vi "FactorPass.vi"(7 "Coordenada bola":dbl[](array[numeric]), 8 "geometry":T6, 9 "Coordenada robo":dbl[](array[numeric]), 10 "enemy_robots":T1[](array[typedef]), 11 "enemy_goalie_id":dbl) -> (0 "id inimigo \nmaior diferença \nde tempo":dbl, 1 "Dif. tempo\ninimigo bola":dbl, 2 "t":dbl, 3 "Critério de marcação Normalizado":dbl, 4 "Robô marcado?":bool=TRUE, 5 "Array out":dbl[][](array[numeric]), 6 "menor dist":dbl)   [LabVIEW 2018]
uses:
  newpass/SSLView/Core/Field Size.ctl
  newpass/SSLView/Core/AI Robot.ctl
  newpass/SSLView/Intel/Functions Enum.ctl
  newpass/SSLView/Intel/AttackerStates.ctl
  newpass/SSLView/Path Planning/RRT/PathDests.ctl
  newpass/SSLView/Path Planning/RRT/PathDest.ctl
  2b1c05b2-3bf1-4219-9740-877ec4118c70.vi
  <vilib>/Array/Sort 2D Array - Pop Stack.vi
  <vilib>/Array/Sort 2D Array - Push Stack.vi
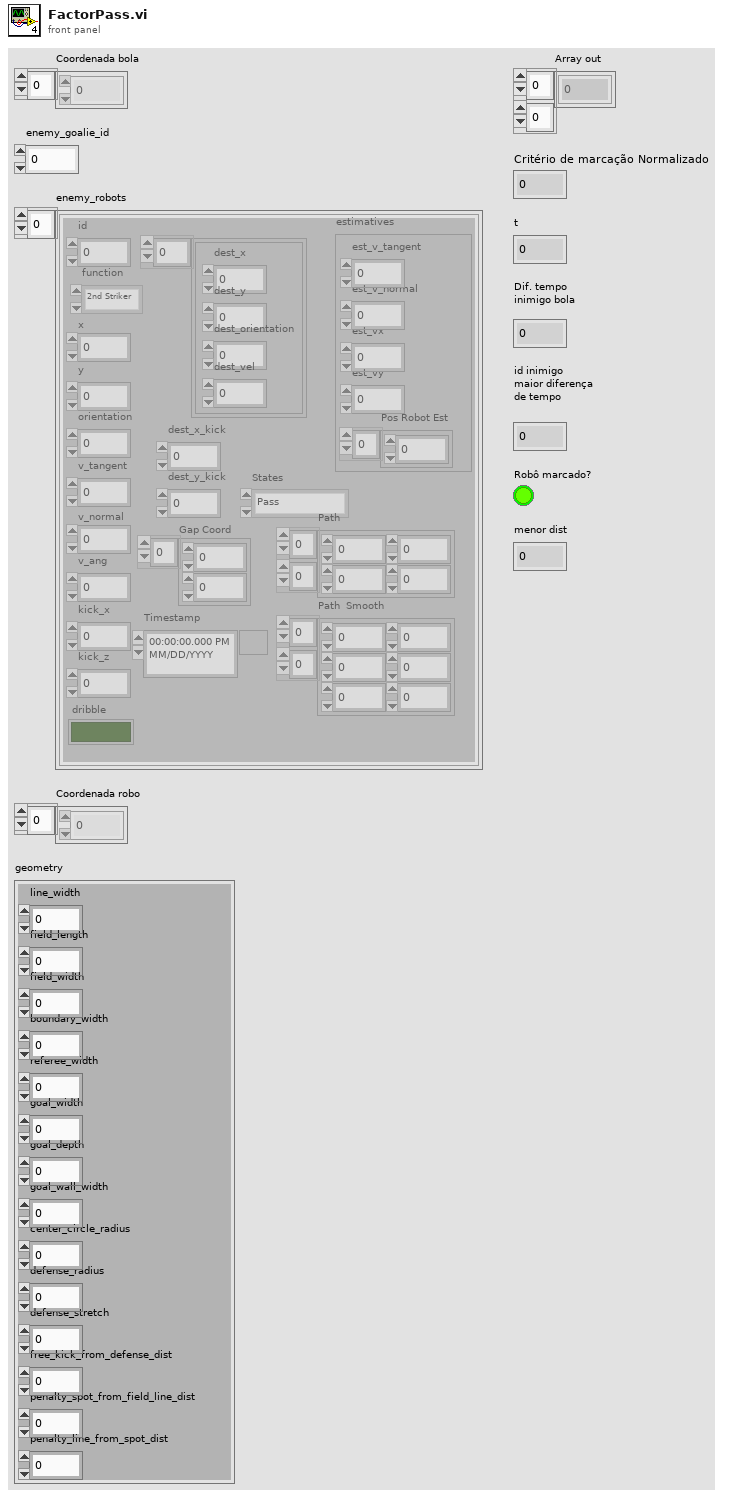
[diagram p1: front panel]
types:
  T1 = typedef "AI Robot.ctl" = cluster{"id":u32, "function":T2, "x":dbl, "y":dbl, "orientation":dbl, "v_tangent":dbl, "v_normal":dbl, "v_ang":dbl, "kick_x":dbl, "kick_z":dbl, "dribble":bool, "Timestamp":timestamp, "estimatives":cluster{"est_v_tangent":dbl, "est_v_normal":dbl, "est_vx":dbl, "est_vy":dbl, "Pos Robot Est":dbl[]}, "dest_x_kick":dbl, "dest_y_kick":dbl, "Gap Coord":dbl[], "States":T3, "Path ":dbl[][], "Path  Smooth":dbl[][], "Dest":T4}
  T2 = typedef "Functions Enum.ctl" = enum16{"2nd Striker", "Attacker", "Goalie", "Defender", "Striker", "Goto 0", "Dummy", "Kicker", "ZigZag 0", "ZigZag 1", "ZigZag 2", "ZigZag 3", "ZigZag 4", "ZigZag 5", "ZigZag 6", "ZigZag 7", "ZigZag 8", ""}
  T3 = typedef "AttackerStates.ctl" = enum16{"Pass", "GoToTangent", "BallGetting", "GoToKick", ""}
  T4 = typedef "PathDests.ctl" = T5[]
  T5 = typedef "PathDest.ctl" = cluster{"dest_x":dbl, "dest_y":dbl, "dest_orientation":dbl, "dest_vel":dbl}
  T6 = typedef "Field Size.ctl" = cluster{"line_width":u32, "field_length":u32, "field_width":u32, "boundary_width":u32, "referee_width":u32, "goal_width":u32, "goal_depth":u32, "goal_wall_width":u32, "center_circle_radius":u32, "defense_radius":u32, "defense_stretch":u32, "free_kick_from_defense_dist":u32, "penalty_spot_from_field_line_dist":u32, "penalty_line_from_spot_dist":u32}
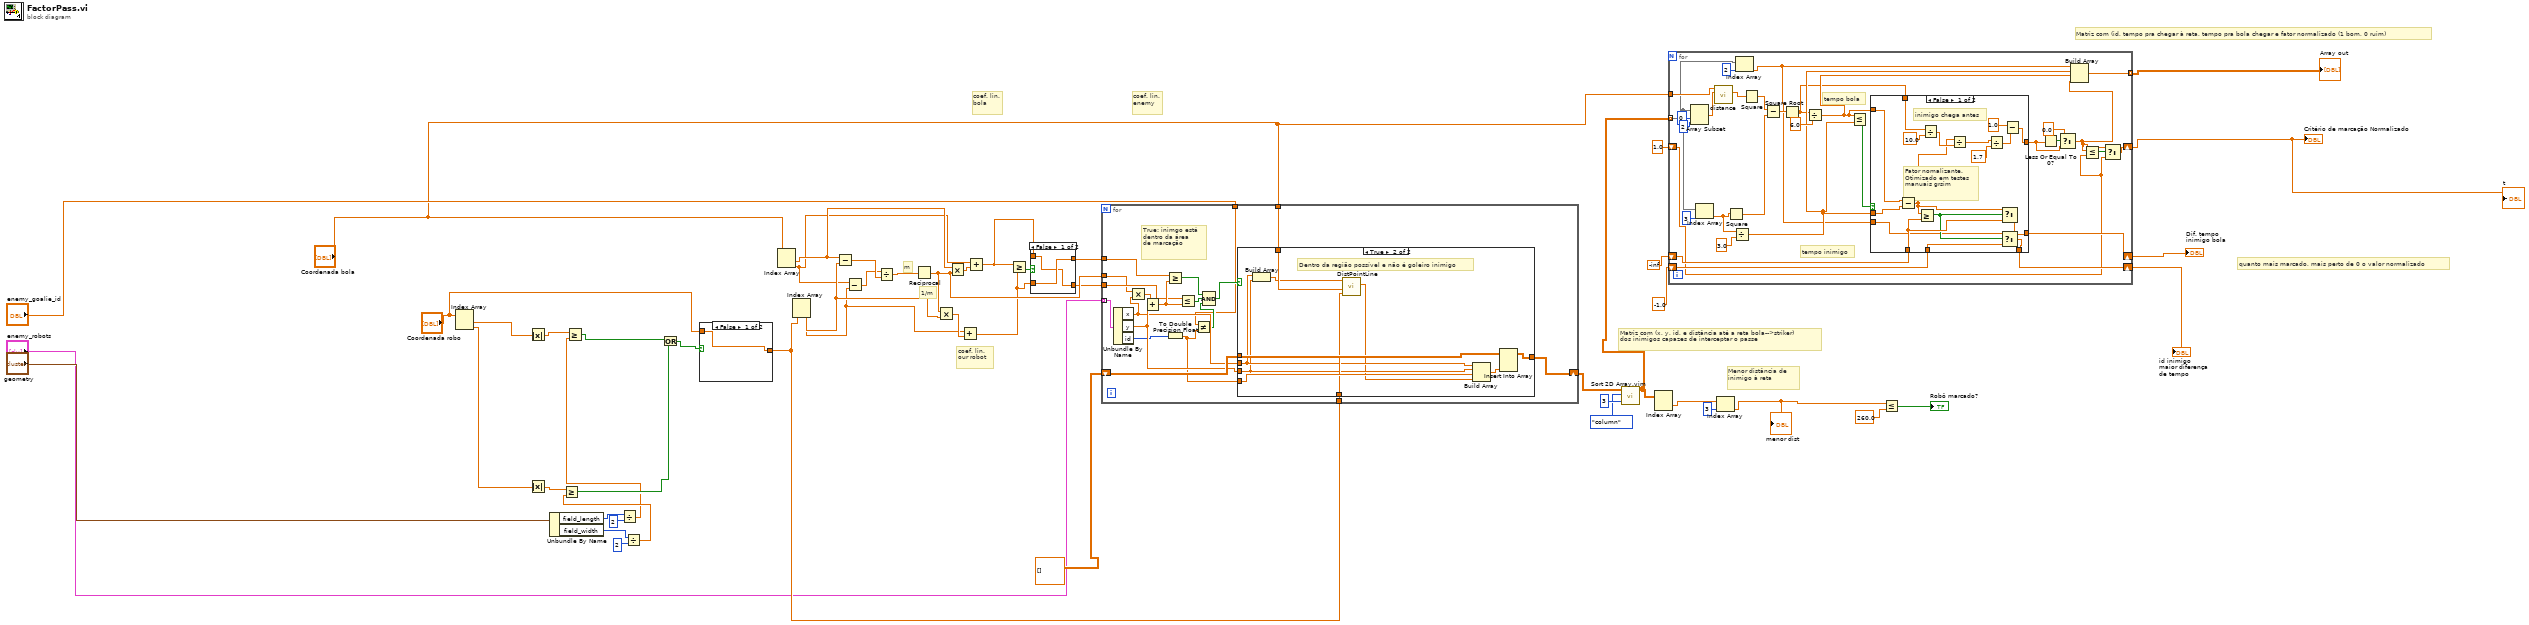
[diagram p0: block diagram]
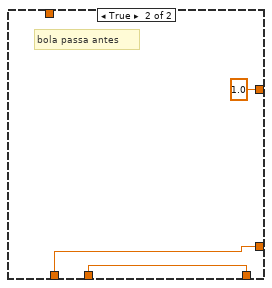
[diagram p2: hidden frame]
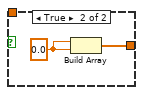
[diagram p3: hidden frame]
diagram:
  # "Matriz com (id, tempo pra chegar à reta, tempo pra bola chegar e fator normalizado (1 bom, 0 ruim)"
  # "quanto mais marcado, mais perto de 0 o valor normalizado"
  # "Menor distância de \ninimigo à reta"
  # "Matriz com (x, y, id, e distância até a reta bola-->striker) \ndos inimigos capazes de interceptar o passe"
  # "coef. lin.\nbola"
  # "coef. lin.\nenemy"
  # "coef. lin.\nour robot"
  # "1/m"
  # "m"
  n1 = Index Array(array="Coordenada robo") -> (element #1=w45:dbl, element #2=w46:dbl)  [unwired: 2 in]
  n2 = Absolute Value(x=w45) -> (abs(x)=w23:dbl)
  n3 = Absolute Value(x=w46) -> (abs(x)=w25:dbl)
  n4 = Unbundle By Name("geometry") -> ("field_length"=w19:u32, "field_width"=w22:u32)
  n5 = Divide(x=w19, y=2) -> (x/y=w24:dbl)
  n6 = Greater Or Equal?(x=w23, y=w24) -> (x >= y?=w27:bool)
  n7 = Divide(x=w22, y=u32 2) -> (x/y=w26:dbl)
  n8 = Greater Or Equal?(x=w25, y=w26) -> (x >= y?=w28:bool)
  n9 = Or(x=w27, y=w28) -> (x .or. y?=w30:bool)
  n10 = case shown="False" w30 {
    tunnel: [w52 w53] -> w31
    tunnel: "Coordenada robo" -> [w52 _]
    frame False {
    }
    frame True {
      w54 = 0.0
      n11 = Build Array(w54, w54) -> (w53:dbl[])
    }
  }
  n12 = Index Array(array="Coordenada bola") -> (element #1=w42:dbl, element #2=w2:dbl)  [unwired: 2 in]
  n13 = Index Array(array=w31) -> (element #1=w41:dbl, element #2=w3:dbl)  [unwired: 2 in]
  n14 = Subtract(x=w42, y=w41) -> (x-y=w5:dbl)
  n15 = Subtract(x=w2, y=w3) -> (x-y=w4:dbl)
  n16 = Divide(x=w4, y=w5) -> (x/y=w1:dbl)
  n17 = Reciprocal(x=w1) -> (1/x=w44:dbl)
  n18 = Multiply(x=w44, y=w41) -> (x*y=w40:dbl)
  n19 = Multiply(x=w42, y=w44) -> (x*y=w43:dbl)
  n20 = Add(x=w3, y=w40) -> (x+y=w9:dbl)
  n21 = Add(x=w2, y=w43) -> (x+y=w8:dbl)
  n22 = Greater Or Equal?(x=w8, y=w9) -> (x >= y?=w7:bool)
  n23 = case shown="False" w7 {
    tunnel: [w56 w58] -> w10
    tunnel: w8 -> [w55 w58]
    tunnel: [w55 w57] -> w11
    tunnel: w9 -> [w56 w57]
    frame False {
    }
    frame True {
    }
  }
  n24 = for {
    tunnel: "enemy_robots" -> [w77] mode=indexing
    tunnel: w44 -> [w65]
    shift-right: [w75] -> w14
    shift-left: dbl[][] [] -> [w76]
    tunnel: w10 -> [w70]
    tunnel: w11 -> [w69]
    tunnel: "Coordenada bola" -> [w67]
    tunnel: w31 -> [w66]
    tunnel: "enemy_goalie_id" -> [w60]
    # "True: inimgo está \ndentro da área\nde marcação"
    n25 = Unbundle By Name(w77) -> ("x"=w64:dbl, "y"=w68:dbl, "id"=w62:u32)
    n26 = Multiply(x=w65, y=w64) -> (x*y=w63:dbl)
    n27 = Add(x=w63, y=w68) -> (x+y=w74:dbl)
    n28 = Greater Or Equal?(x=w70, y=w74) -> (x >= y?=w72:bool)
    n29 = To Double Precision Float(number=w62) -> (double precision float=w59:dbl)
    n30 = Less Or Equal?(x=w69, y=w74) -> (x <= y?=w73:bool)
    n31 = Not Equal?(x=w60, y=w59) -> (x != y?=w61:bool)
    n32 = Compound Arithmetic op=AND(w72, w73, w61) -> (w71:bool)
    n33 = case shown="True" w71 {
      tunnel: w76 -> [w78 w88]
      tunnel: [w78 w87] -> w75
      tunnel: w64 -> [_ w82]
      tunnel: w68 -> [_ w81]
      tunnel: w59 -> [_ w86]
      tunnel: w67 -> [_ w84]
      tunnel: w66 -> [_ w83]
      frame False {
        # "Fora da região possível ou é goleiro inimigo"
      }
      frame True {
        # "Dentro da região possível e não é goleiro inimigo"
        n34 = Build Array(w82, w81) -> (w80:dbl[])
        n35 = call "DistPointLine.vi"("P2"=w83, "P1"=w84, "Q"=w80) -> ("distance"=w79:dbl)  [unwired: 8 in]
        n36 = Build Array(w82, w81, w86, w79) -> (w85:dbl[])
        n37 = Insert Into Array(array=w88, new element=w85) -> (w87:dbl[][])  [unwired: 2 in]
      }
    }
  }
  n38 = call "Sort 2D Array.vim"("index"=3, "dimension to index (column)"=enum16{"column", "row"}."column", "2D array"=w14) -> ("sorted 2D array"=w35:dbl[][])  [unwired: 7 in, 1 out]
  n39 = Index Array(array=w35) -> (element=w33:dbl[])  [unwired: 2 in]
  n40 = for {
    tunnel: "Coordenada bola" -> [w102]
    tunnel: w35 -> [w101] mode=indexing
    shift-right: [w97] -> w48
    shift-left: -inf -> [w107]
    tunnel: [w106] -> w37 mode=indexing
    shift-right: [w100] -> w39
    shift-left: -1.0 ("Numeric") -> [w98]
    shift-right: [w92] -> w50
    shift-left: 1.0 ("t") -> [w90]
    # "tempo inimigo"
    # "tempo bola"
    n41 = Array Subset(array=w101, index=0, length=2) -> (w116:dbl[])
    n42 = Index Array(array=w101, index=3) -> (element=w110:dbl)
    n43 = call "distance.vi"("P1"=w116, "P2"=w102) -> ("Dist P1P2"=w115:dbl)  [unwired: 9 in]
    n44 = Square(x=w110) -> (x^2=w113:dbl)
    n45 = Divide(x=w110, y=3.0) -> (x/y=w104:dbl)
    n46 = Index Array(array=w101, index=2) -> (element=w99:dbl)
    n47 = Square(x=w115) -> (x^2=w114:dbl)
    n48 = Subtract(x=w114, y=w113) -> (x-y=w112:dbl)
    n49 = Square Root(x=w112) -> (sqrt(x)=w96:dbl)
    n50 = Divide(x=w96, y=6.0) -> (x/y=w105:dbl)
    n51 = Less Or Equal?(x=w105, y=w104) -> (x <= y?=w108:bool)
    n52 = case shown="False" w108 {
      tunnel: w104 -> [w134 _]
      tunnel: w105 -> [w135 _]
      tunnel: [w126 w139] -> w97
      tunnel: w107 -> [w136 w139]
      tunnel: [w132 w138] -> w100
      tunnel: w99 -> [w131 _]
      tunnel: w98 -> [w130 w138]
      tunnel: w96 -> [w129 _]
      tunnel: [w121 1.0] -> w94
      frame False {
        # "Fator nomalizante.\nOtimizado em testes\nmanuais grsim"
        # "inimigo chega antes"
        n53 = Subtract(x=w135, y=w134) -> (x-y=w120:dbl)
        n54 = Greater Or Equal?(x=w120, y=w136) -> (x >= y?=w133:bool)
        n55 = Divide(x=w129, y=10.0) -> (x/y=w127:dbl)
        n56 = Divide(x=w120, y=w127) -> (x/y=w125:dbl)
        n57 = Divide(x=w125, y=1.7) -> (x/y=w122:dbl)
        n58 = Select(t=w120, s=w133, f=w136) -> (s? t:f=w126:dbl)
        n59 = Select(t=w131, s=w133, f=w130) -> (s? t:f=w132:dbl)
        n60 = Subtract(x=1.0, y=w122) -> (x-y=w121:dbl)
      }
      frame True {
        # "bola passa antes"
      }
    }
    n61 = Less Or Equal To 0?(x=w94) -> (x <= 0?=w95:bool)
    n62 = Select(t=0.0, s=w95, f=w94) -> (s? t:f=w91:dbl)
    n63 = Build Array(w99, w104, w105, w91) -> (w106:dbl[])
    n64 = Less Or Equal?(x=w91, y=w90) -> (x <= y?=w89:bool)
    n65 = Select(t=w91, s=w89, f=w90) -> (s? t:f=w92:dbl)
  }
  "Dif. tempo\ninimigo bola" <- w48
  "Array out" <- w37
  "id inimigo \nmaior diferença \nde tempo" <- w39
  "Critério de marcação Normalizado" <- w50
  "t" <- w50
  n66 = Index Array(array=w33, index=3) -> (element=w32:dbl)
  "menor dist" <- w32
  n67 = Less Or Equal?(x=w32, y=260.0) -> (x <= y?=→"Robô marcado?":bool)
